vi "SysDef.Search.Parent.vi"(8 "error in (no error)":errorcluster, 11 "nodeID":u64) -> (0 "error out":errorcluster, 1 "Value out":u64, 3 "nodeID out":u64, 4 "Found?":bool)   [LabVIEW 2024, in "Advanced System Definition.lvlib"]
uses:
  SysDef API/Advanced System Definition.lvlib
  C:/NetCore/niveristand-custom-device-development-tools/advanced-sysdef-api/Source/_SubVIs/SysDef.Search.Parent.vi/NationalInstruments.VeriStand.SystemDefinitionAPI
  NationalInstruments.VeriStand.SystemDefinitionAPI
  C:/NetCore/niveristand-custom-device-development-tools/advanced-sysdef-api/Source/_SubVIs/SysDef.Search.Parent.vi/NationalInstruments.VeriStand.SystemStorage
  NationalInstruments.VeriStand.SystemStorage
  <vilib>/NI VeriStand/Custom Device API/Custom Device API.lvlib
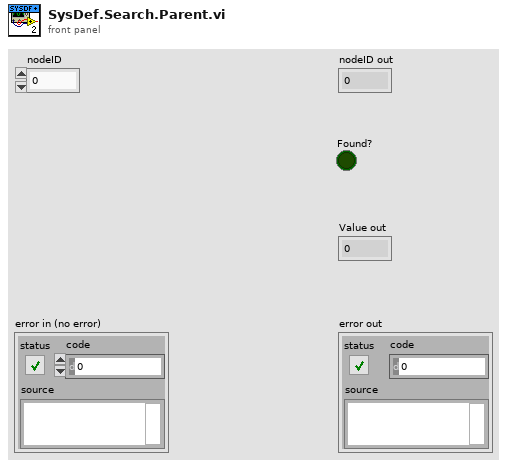
[diagram p1: front panel]
types:
  T1 = typedef "Custom Device API.lvlib/Custom Device Item Ref.ctl" = u64
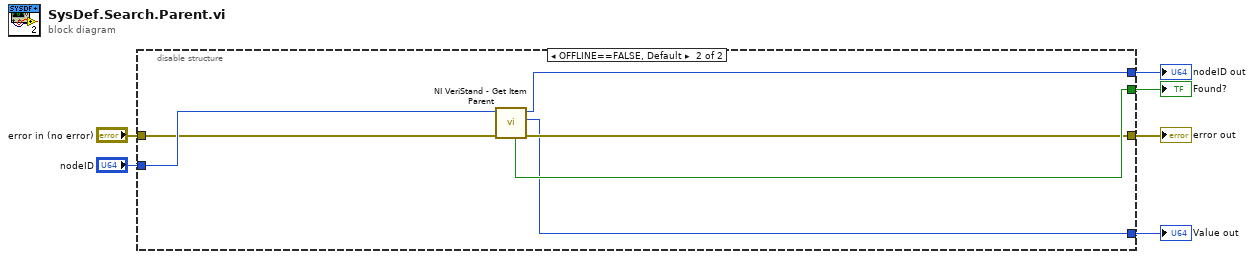
[diagram p0: block diagram]
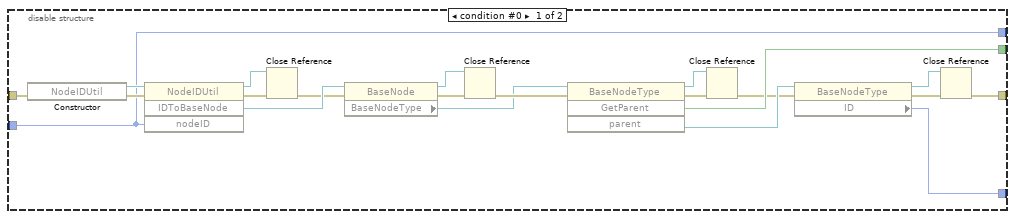
[diagram p2: hidden frame]
diagram:
  n1 = disable-structure shown="OFFLINE==FALSE, Default" {
    disable-tunnel: "error in (no error)" -> [w21 w32]
    disable-tunnel: "nodeID" -> [w17 w33]
    disable-tunnel: [w18 w30] -> w4
    disable-tunnel: [w11 w31] -> w3
    disable-tunnel: [w12 w28] -> w2
    disable-tunnel: [w17 w29] -> w1
    frame condition #0 {
      n2 = constructor class="NodeIDUtil"(error in=w21) -> (reference out=w27:refnum<k24>, error out=w26:errorcluster)  [unwired: 2 in, 1 out]
      n3 = invoke class="NodeIDUtil" method="IDToBaseNode"(reference=w27, error in=w26, "nodeID"=w17) -> (reference out=w22:refnum<k24>, error out=w24:errorcluster, "IDToBaseNode"=w25:refnum<k24>)  [unwired: 1 in, 1 out]
      n4 = Close Reference(reference=w22, error in (no error)=w24) -> (error out=w23:errorcluster)
      n5 = property class="BaseNode"(reference=w25, error in=w23) -> (reference out=w20:refnum<k24>, error out=w19:errorcluster, "BaseNodeType"=w15:refnum<k24>)
      n6 = Close Reference(reference=w20, error in (no error)=w19) -> (error out=w16:errorcluster)
      n7 = invoke class="BaseNodeType" method="GetParent"(reference=w15, error in=w16) -> (reference out=w9:refnum<k24>, error out=w10:errorcluster, "GetParent"=w11:bool, "parent"=w8:refnum<k24>)  [unwired: 2 in]
      n8 = Close Reference(reference=w9, error in (no error)=w10) -> (error out=w7:errorcluster)
      n9 = property class="BaseNodeType"(reference=w8, error in=w7) -> (reference out=w14:refnum<k24>, error out=w13:errorcluster, "ID"=w12:u64)
      n10 = Close Reference(reference=w14, error in (no error)=w13) -> (error out=w18:errorcluster)
    }
    frame condition #1 (active) {
      n11 = call <vilib>:"NI VeriStand - Get Item Parent.vi"("error in (no error)"=w32, "Item Ref in"=w33) -> ("error out"=w30:errorcluster, "Parent Ref"=w28:T1, "Item Ref out"=w29:T1, "Found"=w31:bool)  [unwired: 6 in]
    }
  }
  "nodeID out" <- w1
  "error out" <- w4
  "Value out" <- w2
  "Found?" <- w3
